vi "ResonanceAnalyzer.vi"() -> ()   [LabVIEW 2014]
uses:
  <vilib>/imath/engines/lvmath2/RunTimeEngine/Managers/WorkSpace/UID Generator.vi
  <vilib>/imath/engines/lvmath2/RunTimeEngine/RangeToken/NIMS_Range.vi
  <vilib>/imathl/engines/lvmath/Functions/Error Handling/Create Error.vi
  <vilib>/imath/engines/lvmath2/RunTimeEngine/LocalVariableDefStatement/MC_LocalVariableDefStatement_Display.vi
  <vilib>/imath/engines/lvmath2/RunTimeEngine/RunTimeType/NIMS_RunTimeType_From StrictType (excl LVString).vi
  <vilib>/imath/engines/lvmath2/RunTimeEngine/ArithmeticOperatorToken/NIMS_ArithmeticOperator_minus.vi
  <vilib>/imath/engines/lvmath2/RunTimeEngine/BuiltInFunctions/size/NIMS_I32Row=size(GRow).vi
  <vilib>/imath/engines/lvmath2/RunTimeEngine/BuiltInFunctions/randnormal/NIMS_randnormal(I32V).vi
  <vilib>/imath/engines/lvmath2/RunTimeEngine/ErrorHandling/NIMS_Create Error From Enums.vi
  <vilib>/imath/engines/lvmath2/RunTimeEngine/ArithmeticOperatorToken/NIMS_ArithmeticOperator_plus.vi
  <vilib>/imath/engines/lvmath2/RunTimeEngine/NodeEndStatement/NIMS_NodeEndStatement_Get Vector.vi
  <vilib>/imath/engines/lvmath2/RunTimeEngine/Managers/SymbolTable/Clear UID.vi
  <vilib>/imath/engines/lvmath2/RunTimeEngine/Managers/SymbolTable/NIMS_WorkSpace.lvlib
  <vilib>/imath/engines/lvmath/Functions/Error Handling/MergeErrorsWrapper.vi
  <vilib>/imath/engines/lvmath2/RunTimeEngine/NodeEndStatement/NIMS_NodeEndStatement_Output.vi
  <vilib>/imath/engines/lvmath2/RunTimeEngine/ErrorHandling/NIMS_Finalize Error.vi
panel:
  out "Best-fit Parameters, Q and Center Freq.":waveform(dbl)={"t0"=timestamp(0 s since 1904-01-01), "dt"=1.0, "Y"=[10.003799287811958, 599.9384641338464], "attributes"=variant("NI_ChannelName"=variant(string "Best Fit Coefficients"))}
  out "XY Graph":cluster{"all rows":dbl[], "all rows":dbl[]}(graph)={"all rows"=[400.0, 405.0, 410.0, 415.0, 420.0, 425.0, 430.0, 435.0, 440.0, 445.0, 450.0, 455.0, 460.0, 465.0, 470.0, 475.0, 480.0, 485.0, 490.0, 495.0, 500.0, 505.0, 510.0, 515.0, 520.0, 525.0, 530.0, 535.0, 540.0, 545.0, 550.0, 555.0, 560.0, 565.0, 570.0, 575.0, 580.0, 585.0, 590.0, 595.0, 600.0, 605.0, 610.0, 615.0, 620.0, 625.0, 630.0, 635.0, 640.0, 645.0, 650.0, 655.0, 660.0, 665.0, 670.0, 675.0, 680.0, 685.0, 690.0, 695.0, 700.0, 705.0, 710.0, 715.0, 720.0, 725.0, 730.0, 735.0, 740.0, 745.0, 750.0, 755.0, 760.0, 765.0, 770.0, 775.0, 780.0, 785.0, 790.0, 795.0, 800.0], "all rows"=[0.14179461511558822, 0.11996062497552826, 0.10860337049693136, 0.13697578852440553, 0.125205952546278, 0.15087920725809642, 0.1503491525700989, 0.1441004560201708, 0.156308701198372, 0.14624062139124644, 0.17081095115873793, 0.16603906357041662, 0.20059545082090907, 0.18919831169838094, 0.19231379222713355, 0.19608486183058946, 0.23900913519857123, 0.23349924239309108, 0.24377867471378445, 0.24093086111064138, 0.26371580527304855, 0.26793633239921977, 0.2941727912598759, 0.30422665055310694, 0.31635476419709446, 0.33199964853399055, 0.37347439570600943, 0.39589632517242895, 0.43385046653369697, 0.45691523717339283, 0.5009897089079943, 0.5415315358777776, 0.585008508335163, 0.6363765579061614, 0.7044067126031366, 0.7726340799581203, 0.8282859544101132, 0.9036148081425924, 0.9523639150338892, 0.9711080260119477, 1.0057599570511802, 0.9884107925276422, 0.9486052548976953, 0.9096819220690453, 0.8484032734683263, 0.7534300597428925, 0.7227919489492753, 0.6574836994405368, 0.609858783485813, 0.5724295985484753, 0.5277343260871714, 0.480937212931507, 0.45138975112357305, 0.43455561332905723, 0.41616229803959776, 0.39746803193752206, 0.3554048541430116, 0.3549803755212468, 0.34412742537274404, 0.32152754465975336, 0.3059023150832531, 0.2970206297360512, 0.2830237232036178, 0.29323512722191125, 0.2442930428401266, 0.24997963354563502, 0.24347245033074158, 0.25413549097009225, 0.23373026496041063, 0.22619515936320245, 0.23426401252085732, 0.212845302052927, 0.20596955412624793, 0.2085869831035697, 0.20220110197050484, 0.18625539237279165, 0.19818146759337868, 0.16087337999081203, 0.17009831951310145, 0.17687533070394046, 0.16801278086965266]}
  in  "Tab Control":enum32{"Simulation", "Experiment"}(tab)
  in  "Q":i32=10
  in  "Center Frequency":i32=600
  in  "Start Frequency":i32=400
  in  "End Frequency":i32=800
  in  "df":i32=5
  in  "Noise Level":dbl=0.01
  in  "Path":path=path "U:/phys 434/week5/600to800detailDataSpreadsheet"
  # "Q approximation"
  # "Center Freq. approximation"
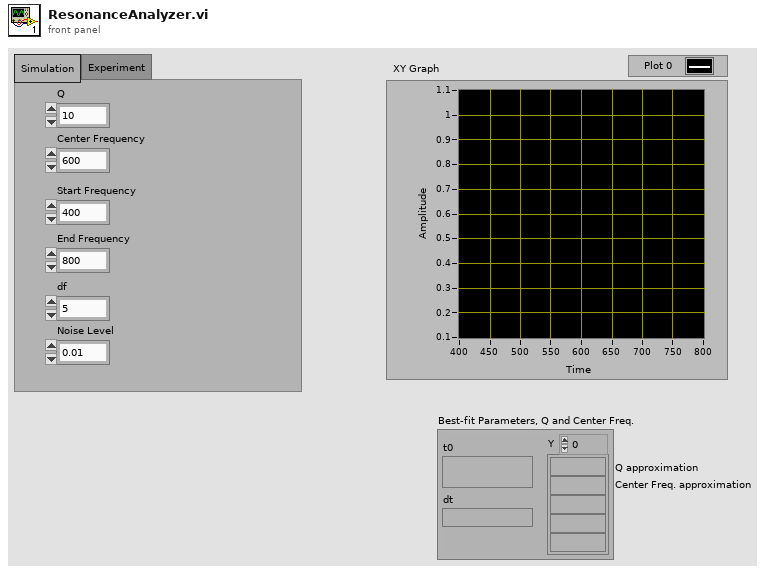
[diagram p1: front panel]
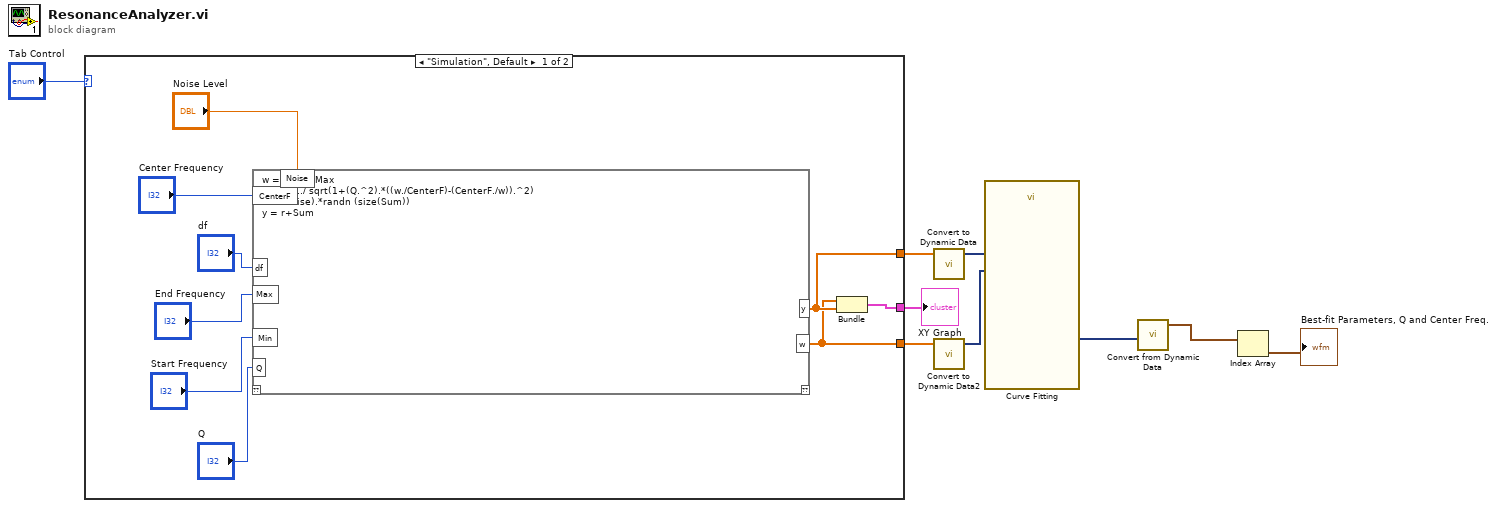
[diagram p0: block diagram]
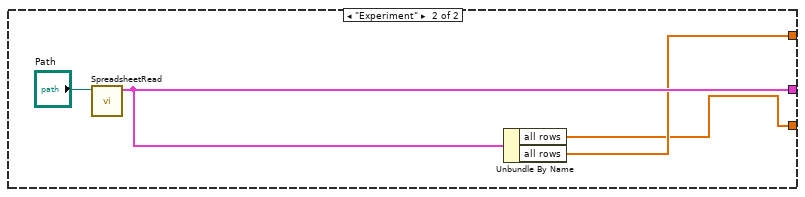
[diagram p2: hidden frame]
diagram:
  n1 = case shown="\"Simulation\", Default" "Tab Control" {
    tunnel: [w12 w181] -> w8
    tunnel: [w11 w180] -> w7
    tunnel: [w10 w179] -> w4
    frame "Simulation", Default {
      n2 = mathscript code="w = Min:df:Max\nSum =1./ sqrt(1+(Q.^2).*((w./CenterF)-(CenterF./w)).^2)\nr = (Noise).*randn (size(Sum))\ny = r+Sum"("Min"="Start Frequency", "Max"="End Frequency", "df"="df", "Q"="Q", "CenterF"="Center Frequency", "Noise"="Noise Level") -> ("y"=w11:dbl[], "w"=w10:dbl[])  [unwired: 1 in, 1 out]
      n3 = Bundle("w"=w10, "y"=w11) -> (w12:cluster{"w":dbl[], "y":dbl[]})  [unwired: 1 in]
    }
    frame "Experiment" {
      n4 = call "SpreadsheetRead.vi"("Path"="Path") -> ("XY Graph"=w181:cluster{"all rows":dbl[], "all rows":dbl[]})  [unwired: 10 in]
      n5 = Unbundle By Name(w181) -> ("all rows"=w179:dbl[], "all rows"=w180:dbl[])
    }
  }
  "XY Graph" <- w8
  n6 = call "Convert to Dynamic Data"("Array"=w7) -> ("Dynamic Data Type"=w6:dynamicdata)  [unwired: 3 in]
  n7 = call "Convert to Dynamic Data2"("Array"=w4) -> ("Dynamic Data Type"=w5:dynamicdata)  [unwired: 3 in]
  n8 = call "Curve Fitting"("Locations"=w5, "Signals"=w6) -> ("non-linear coefficients"=w3:dynamicdata)  [unwired: 5 in, 4 out]
  n9 = call "Convert from Dynamic Data"("Dynamic Data Type"=w3) -> ("Array of Waveform"=w2:waveform(dbl)[])  [unwired: 3 in]
  n10 = Index Array(array=w2) -> (element=→"Best-fit Parameters, Q and Center Freq.":waveform(dbl))  [unwired: 1 in]
